vi "DataSort.vi"(11 "DataIn":sgl[](array[numeric])) -> (2 "DataOut":sgl[](array[numeric]), 3 "IndexOut":i32[](array[numeric]))   [LabVIEW 2020]
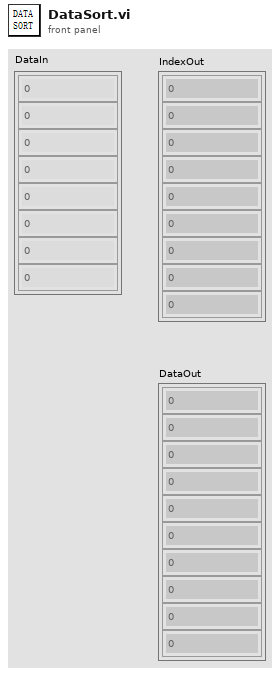
[diagram p1: front panel]
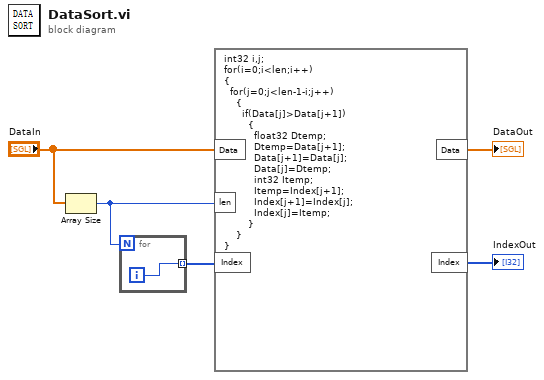
[diagram p0: block diagram]
diagram:
  n1 = Array Size(array="DataIn") -> (size(s)=w3:i32)
  n2 = for {
    N: w3 -> [_]
    tunnel: [w6] -> w2 mode=indexing
    i -> [w6]
  }
  n3 = formula code="int32 i,j;\nfor(i=0;i<len;i++)\n{\n  for(j=0;j<len-1-i;j++)\n    {\n      if(Data[j]>Data[j+1])\n        {\n          float32 Dtemp;\n          Dtemp=Data[j+1];\n          Data[j+1]=Data[j];\n          Data[j]=Dtemp;\n          int32 Itemp;\n          Itemp=Index[j+1];\n          Index[j+1]=Index[j];\n          Index[j]=Itemp;\n        }\n    }\n}" ("公式节点")("Data"="DataIn", "len"=w3, "Index"=w2) -> ("Data"=→"DataOut":sgl[], "Index"=→"IndexOut":i32[])
